vi "Target Colour Testing.vi"() -> ()   [LabVIEW 2013]
uses:
  <vilib>/Rock Robotics/WPI/Camera/WPI_CameraSettings Read MJPG.ctl
  <vilib>/Rock Robotics/WPI/Camera/WPI_CameraImageSize.ctl
  <vilib>/vision/Measure.llb/Edge Options.ctl
  <vilib>/vision/Measure.llb/Edge Polarity.ctl
  <vilib>/vision/Measure.llb/Straight Edge Options.ctl
  <vilib>/vision/Measure.llb/Straight Edge Process.ctl
  <vilib>/vision/NI_Vision_Development_Module.lvlib
panel:
  out "Threshold Image":T1(plugin-control)
  in  "Blue or Luminance":cluster{i32, i32}(slide)={162, 255} scale=0.0..255.0
  in  "Green or Saturation":cluster{i32, i32}(slide)={12, 255} scale=0.0..255.0
  in  "Threshold Color Mode":enum32{"RGB", "HSL"}(radio)=enum."HSL"
  in  "Red or Hue":cluster{i32, i32}(slide)={119, 182} scale=0.0..255.0
  in  "Edge Options 2":T2={"Edge Polarity"=0, "Kernel Size"=3, "Width"=3, "Minimum Edge Strength"=10.0, "Interpolation Type"=enum."Bilinear Fixed", "Data Processing Method"=enum."Average"} {"Edge Polarity" items=["All Edges", "Rising Edges", "Falling Edges"]; "Minimum Edge Strength" format="%.2f"; "Width" step=2; "Kernel Size" step=2}
  in  "Line Options 2":T4={"Number of Lines"=2, "Type"=enum."Best Edge Projection", "Min. Score"=10.0, "Max. Score"=1000.0, "Orientation"=0.0, "Angle Range"=10.0, "Angle Tolerance"=1.0, "Step Size"=3, "Min. SNR (db)"=0.0, "Min. Points (%)"=25.0, "Hough Iterations"=5} {"Min. Points (%)" min=0.0 max=100.0; "Min. SNR (db)" min=0.0; "Max. Score" min=0.0 max=1024.0; "Min. Score" min=0.0 max=1024.0 step=1.0}
  in  "Line Options":T4={"Number of Lines"=2, "Type"=enum."Best Edge Projection", "Min. Score"=10.0, "Max. Score"=1000.0, "Orientation"=0.0, "Angle Range"=10.0, "Angle Tolerance"=1.0, "Step Size"=3, "Min. SNR (db)"=0.0, "Min. Points (%)"=25.0, "Hough Iterations"=5} {"Min. Points (%)" min=0.0 max=100.0; "Min. SNR (db)" min=0.0; "Max. Score" min=0.0 max=1024.0; "Min. Score" min=0.0 max=1024.0 step=1.0}
  in  "Edge Options":T2={"Edge Polarity"=0, "Kernel Size"=3, "Width"=3, "Minimum Edge Strength"=10.0, "Interpolation Type"=enum."Bilinear Fixed", "Data Processing Method"=enum."Average"} {"Edge Polarity" items=["All Edges", "Rising Edges", "Falling Edges"]; "Minimum Edge Strength" format="%.2f"; "Width" step=2; "Kernel Size" step=2}
  in  "stop":bool
  in  "Camera Settings":T6={"fps"=15, "compression"=5, "Image Size"=enum."320x240"}
  in  "Camera IP":string="10.40.1.11"
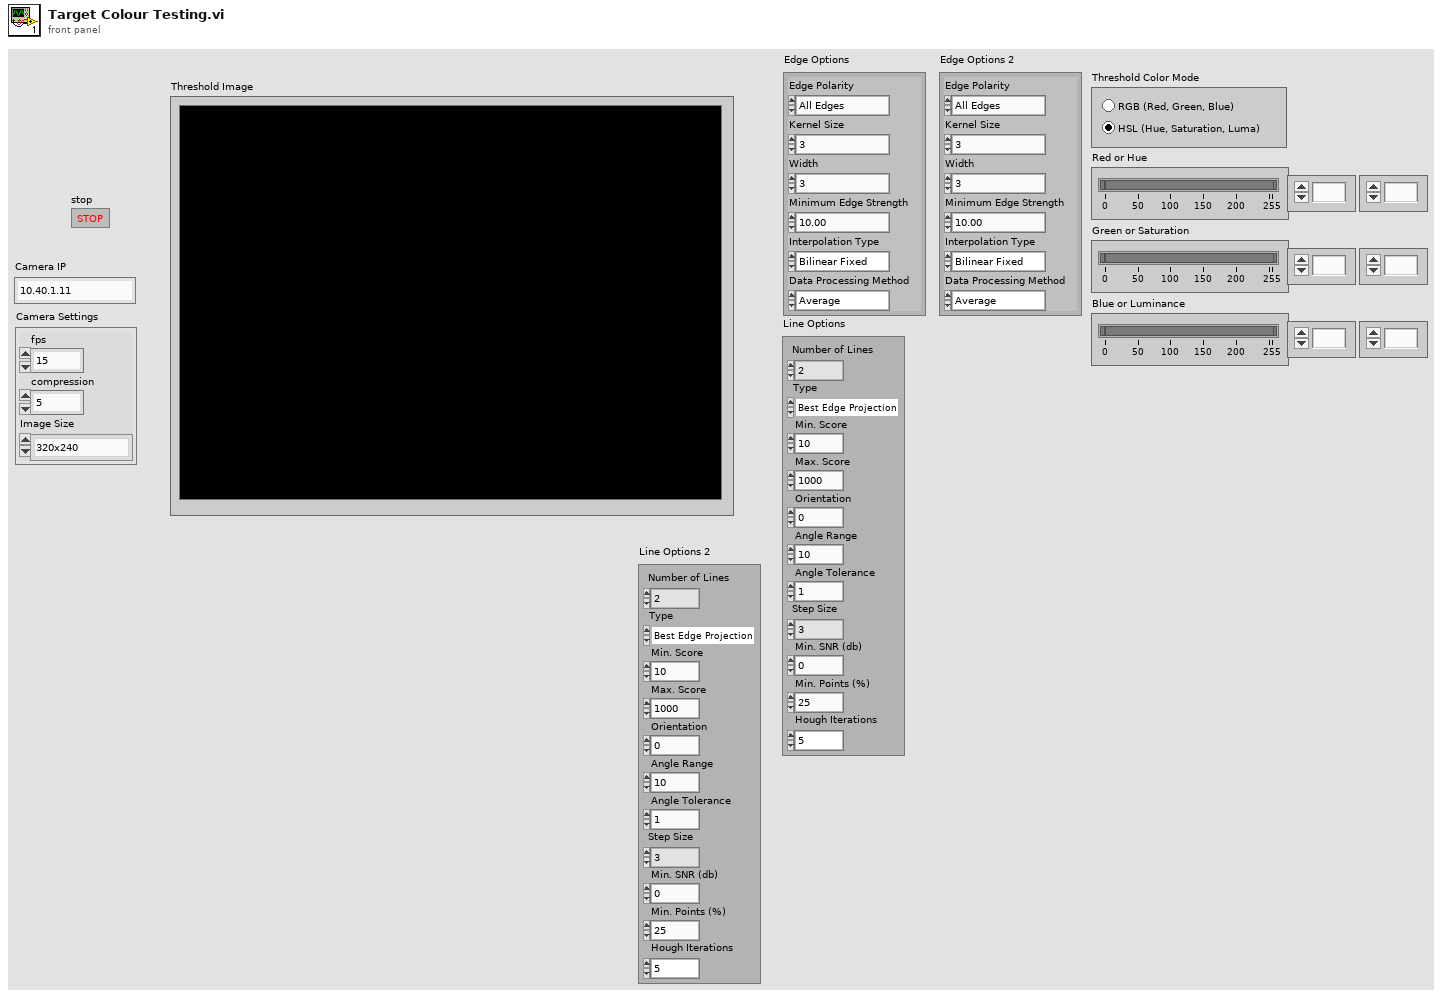
[diagram p1: front panel]
types:
  T1 = typedef "IMAQ Image.ctl" = refnum<image>
  T2 = typedef "Edge Options.ctl" = cluster{"Edge Polarity":T3, "Kernel Size":u32, "Width":u32, "Minimum Edge Strength":sgl, "Interpolation Type":enum32{"Zero Order", "Bilinear", "Quadratic", "Cubic", "Bilinear Fixed"}, "Data Processing Method":enum32{"Average", "Median"}}
  T3 = typedef "Edge Polarity.ctl" = u32
  T4 = typedef "Straight Edge Options.ctl" = cluster{"Number of Lines":i32, "Type":T5, "Min. Score":dbl, "Max. Score":dbl, "Orientation":dbl, "Angle Range":dbl, "Angle Tolerance":dbl, "Step Size":u32, "Min. SNR (db)":dbl, "Min. Points (%)":dbl, "Hough Iterations":i32}
  T5 = typedef "Straight Edge Process.ctl" = enum32{"First Edge Rake", "Best Edge Rake", "Hough Edge Rake", "First Edge Projection", "Best Edge Projection"}
  T6 = typedef "WPI_CameraSettings Read MJPG.ctl" = cluster{"fps":i32, "compression":i32, "Image Size":T7}
  T7 = typedef "WPI_CameraImageSize.ctl" = enum16{"640x480", "320x240", "160x120"}
  T8 = typedef "Image Type" = u32
  T9 = typedef "IMAQ Rectangle" = cluster{"Left":i32, "Top":i32, "Right":i32, "Bottom":i32, "Rotation":dbl}
  T10 = typedef "ROI Descriptor" = cluster{"Global Rectangle":i32[], "Contours":cluster{"ID":enum32{"External", "Internal"}, "Type":u32, "Coordinates":i32[]}[]}
  T11 = cluster{"Global Rectangle":i32[], "Contours":cluster{"Contour Type":u32, "ROI Type":u32, "Points":i32[]}[]}
  T12 = cluster{"Point1 (Pixels)":cluster{"X":sgl, "Y":sgl}, "Point2 (Pixels)":cluster{"X":sgl, "Y":sgl}, "Point1 (Real-World)":cluster{"X":sgl, "Y":sgl}, "Point2 (Real-World)":cluster{"X":sgl, "Y":sgl}, "Angle (Pixel)":dbl, "Angle (Real-World)":dbl, "Score":dbl, "Straightness":dbl, "Average SNR (db)":dbl, "Calibration Valid":bool}[]
  T13 = cluster{"Point1 (Pixels)":cluster{"X":sgl, "Y":sgl}, "Point2 (Pixels)":cluster{"X":sgl, "Y":sgl}, "Point1 (Real-World)":cluster{"X":sgl, "Y":sgl}, "Point2 (Real-World)":cluster{"X":sgl, "Y":sgl}, "Angle (Pixel)":dbl, "Angle (Real-World)":dbl, "Score":dbl, "Straightness":dbl, "Average SNR (db)":dbl, "Calibration Valid":bool}
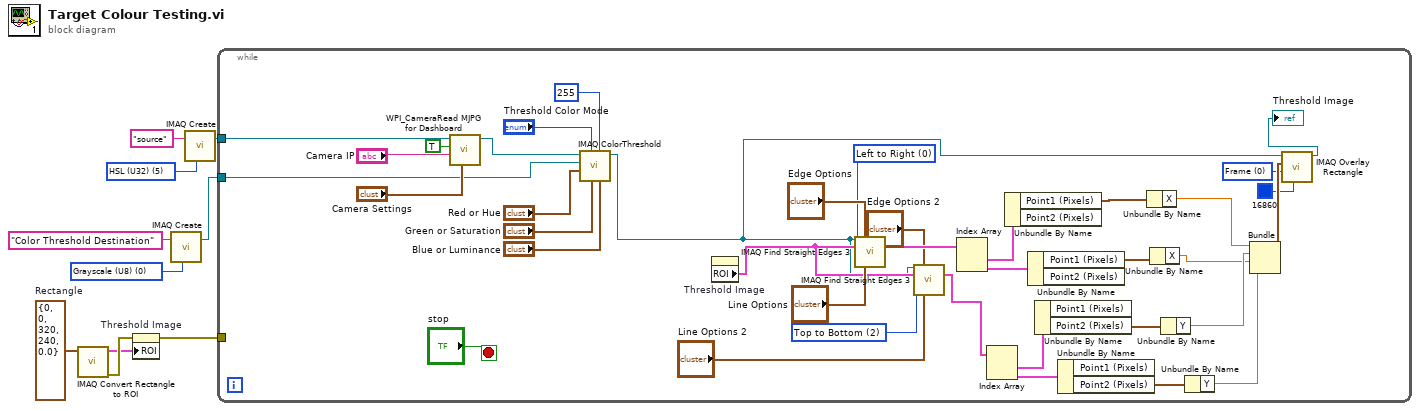
[diagram p0: block diagram]
diagram:
  w4 = T8 0 items=["Grayscale (U8)", "Grayscale (I16)", "Grayscale (SGL)", "Complex (CSG)", "RGB (U32)", "HSL (U32)", "RGB (U64)", "Grayscale (U16)"] ("Image Type")
  w7 = T9 {"Left"=0, "Top"=0, "Right"=320, "Bottom"=240, "Rotation"=0.0}  # Rectangle
  w8 = T8 5 items=["Grayscale (U8)", "Grayscale (I16)", "Grayscale (SGL)", "Complex (CSG)", "RGB (U32)", "HSL (U32)", "RGB (U64)", "Grayscale (U16)"] ("Image Type")
  n1 = call "IMAQ Convert Rectangle to ROI"("Rectangle"=w7) -> ("error out"=w6:errorcluster, "ROI Descriptor"=w5:T10)  [unwired: 8 in]
  n2 = property on="Threshold Image" class="ImageControl"(error in=w6, "ROI"=w5) -> (error out=w1:errorcluster)  [unwired: 1 in, 1 out]
  n3 = call "IMAQ Create"("Image Name"="Color Threshold Destination", "Image Type"=w4) -> ("New Image"=w3:T1)  [unwired: 3 in, 1 out]
  n4 = call "IMAQ Create"("Image Name"="source", "Image Type"=w8) -> ("New Image"=w9:T1)  [unwired: 3 in, 1 out]
  n5 = while {
    tunnel: w9 -> [w44]
    tunnel: w3 -> [w15]
    tunnel: w1 -> [_]
    stop <- "stop" stop-if-true
    w20 = u32 0 items=["Frame", "Fill", "Highlight"] ("Drawing Mode (Frame)")
    w41 = u32 0 items=["Left to Right", "Right to Left", "Top to Bottom", "Bottom to Top"] ("Search Direction")
    w39 = u32 2 items=["Left to Right", "Right to Left", "Top to Bottom", "Bottom to Top"] ("Search Direction")
    n6 = call <vilib>:"WPI_CameraRead MJPG for Dashboard.vi"("Camera Settings"="Camera Settings", "Camera IP"="Camera IP", "Enable"=TRUE, "Refnum in"=w44) -> ("Refnum out"=w14:T1)  [unwired: 4 in, 3 out]
    n7 = call "IMAQ ColorThreshold"("Blue or Luma or Val or Inten Range"="Blue or Luminance", "Replace Value"=255, "Green or Sat Range"="Green or Saturation", "Color Mode"="Threshold Color Mode", "Red or Hue Range"="Red or Hue", "Image Dst"=w15, "Image Src"=w14) -> ("Image Dst Out"=w12:T1)  [unwired: 3 in, 1 out]
    n8 = property on="Threshold Image" class="ImageControl"() -> ("ROI"=w40:T11)  [unwired: 2 in, 2 out]
    n9 = call "IMAQ Find Straight Edges 3"("Image"=w12, "Edge Options"="Edge Options", "ROI Descriptor"=w40, "Search Direction"=w41, "Line Options"="Line Options") -> ("Straight Edges"=w37:T12)  [unwired: 6 in, 4 out]
    n10 = call "IMAQ Find Straight Edges 3"("Image"=w12, "Edge Options"="Edge Options 2", "ROI Descriptor"=w40, "Search Direction"=w39, "Line Options"="Line Options 2") -> ("Straight Edges"=w32:T12)  [unwired: 6 in, 4 out]
    n11 = Index Array(array=w37) -> (element #1=w36:T13, element #2=w35:T13)  [unwired: 2 in]
    n12 = Index Array(array=w32) -> (element #1=w34:T13, element #2=w33:T13)  [unwired: 2 in]
    n13 = Unbundle By Name(w36) -> ("Point1 (Pixels)"=w31:cluster{"X":sgl, "Y":sgl})  [unwired: 1 out]
    n14 = Unbundle By Name(w35) -> ("Point1 (Pixels)"=w30:cluster{"X":sgl, "Y":sgl})  [unwired: 1 out]
    n15 = Unbundle By Name(w34) -> ("Point2 (Pixels)"=w28:cluster{"X":sgl, "Y":sgl})  [unwired: 1 out]
    n16 = Unbundle By Name(w33) -> ("Point2 (Pixels)"=w29:cluster{"X":sgl, "Y":sgl})  [unwired: 1 out]
    n17 = Unbundle By Name(w31) -> ("X"=w27:sgl)
    n18 = Unbundle By Name(w30) -> ("X"=w25:sgl)
    n19 = Unbundle By Name(w28) -> ("Y"=w26:sgl)
    n20 = Unbundle By Name(w29) -> ("Y"=w24:sgl)
    n21 = Bundle("X"=w27, "Y"=w26, "X"=w25, "Y"=w24) -> (w23:cluster{"X":sgl, "Y":sgl, "X":sgl, "Y":sgl})  [unwired: 1 in]
    n22 = call "IMAQ Overlay Rectangle"("Color"=u32 16860, "Drawing Mode (Frame)"=w20, "Rectangle"=w23, "Image"=w12) -> ("Image Out"=→"Threshold Image":T1)  [unwired: 6 in, 1 out]
  }
